vi "pseudoGellermann.vi"(11 "N":i32=10 min=10) -> (3 "Array":bool[](array[boolean]))   [LabVIEW 2013]
panel:
  out "Iterations":i32
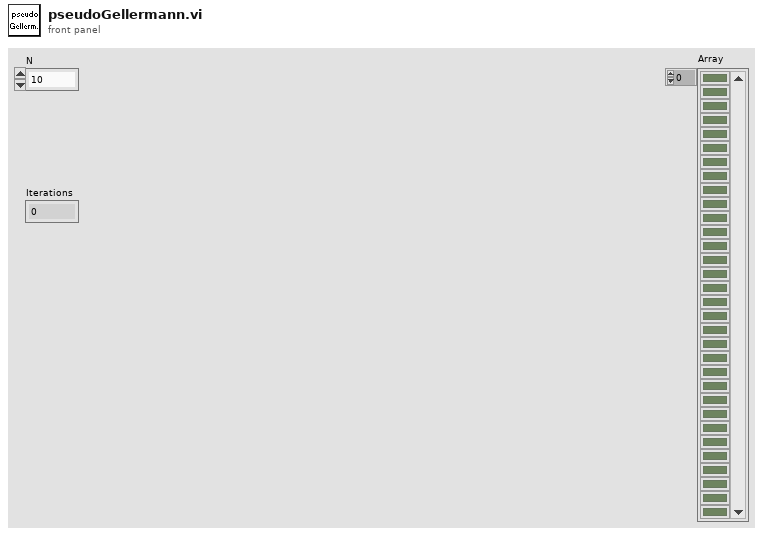
[diagram p1: front panel]
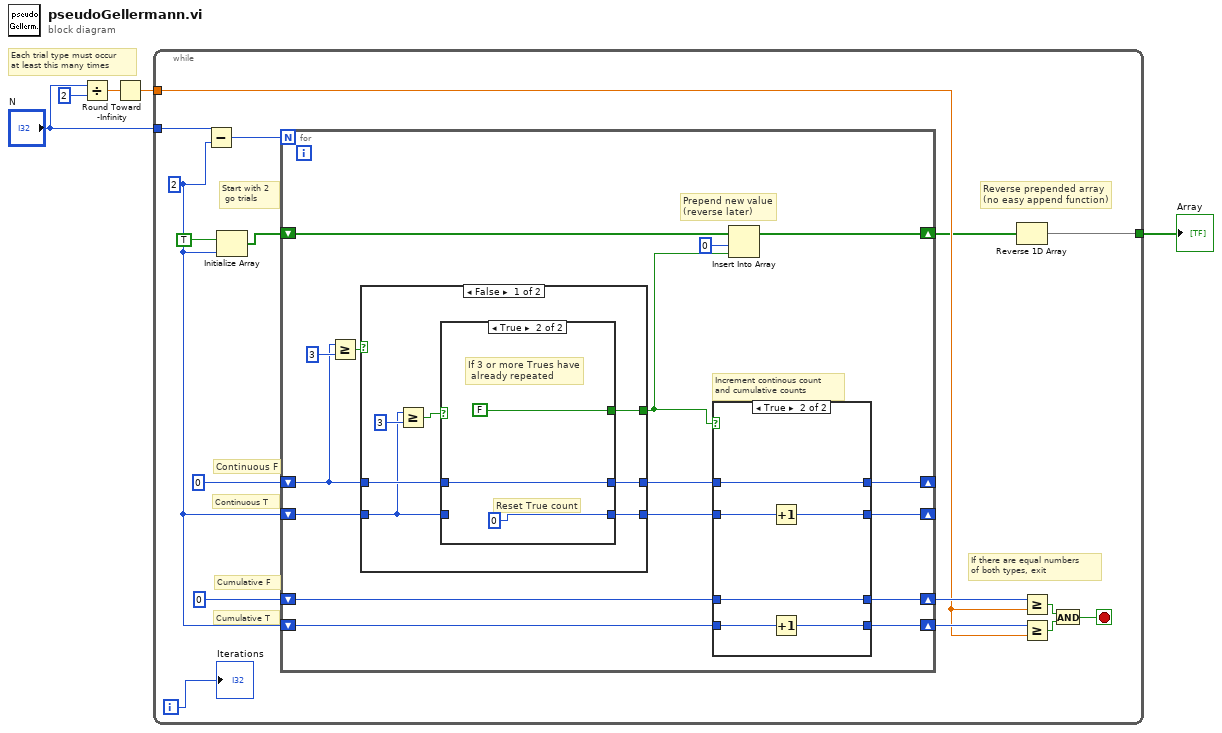
[diagram p0: block diagram]
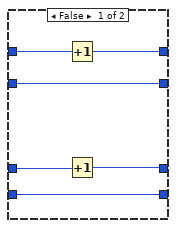
[diagram p2: hidden frame]
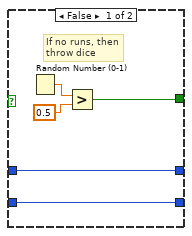
[diagram p3: hidden frame]
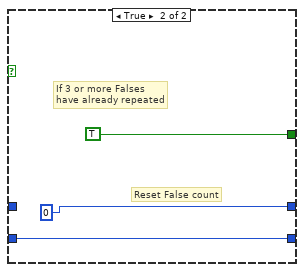
[diagram p4: hidden frame]
diagram:
  # "Each trial type must occur\nat least this many times"
  n1 = Divide(x="N", y=2) -> (x/y=w4:dbl)
  n2 = Round Toward -Infinity(1:w4) -> (0:w2:dbl)
  n3 = while {
    tunnel: "N" -> [w17]
    tunnel: w2 -> [w13]
    tunnel: [w8] -> w1
    i -> [w9]
    stop <- w10 stop-if-true
    w6 = 2 ("dimension size")
    # "Reverse prepended array\n(no easy append function)"
    # "If there are equal numbers\nof both types, exit"
    # "Cumulative T"
    # "Cumulative F"
    # "Start with 2\n go trials"
    # "Continuous T"
    # "Continuous F"
    n4 = Subtract(x=w17, y=w6) -> (x-y=w16:i32)
    n5 = Initialize Array(TRUE, w6) -> (w19:bool[])
    n6 = for {
      N: w16 -> [_]
      shift-right: [w23] -> _
      shift-left: 0 ("dimension size") -> [w35]
      shift-right: [w25] -> _
      shift-left: w6 -> [w34]
      shift-right: [w31] -> w7
      shift-left: w19 -> [w33]
      shift-right: [w28] -> w15
      shift-left: 0 ("dimension size") -> [w30]
      shift-right: [w27] -> w14
      shift-left: w6 -> [w29]
      # "Increment continous count\nand cumulative counts"
      # "Prepend new value\n(reverse later)"
      n7 = Greater Or Equal?(x=w35, y=3) -> (x >= y?=w37:bool)
      n8 = case shown="False" w37 {
        tunnel: w35 -> [w54 _]
        tunnel: w34 -> [w50 w66]
        tunnel: [w53 w66] -> w26
        tunnel: [w52 0 ("dimension size")] -> w24
        tunnel: [w51 TRUE] -> w22
        frame False {
          n9 = Greater Or Equal?(x=w50, y=3) -> (x >= y?=w55:bool)
          n10 = case shown="True" w55 {
            tunnel: w54 -> [w58 w63]
            tunnel: [w57 0 ("dimension size")] -> w53
            tunnel: [w58 w63] -> w52
            tunnel: [w59 FALSE] -> w51
            tunnel: w50 -> [w57 _]
            frame False {
              # "If no runs, then\nthrow dice"
              n11 = Random Number (0-1)() -> (number: 0 to 1=w61:dbl)
              n12 = Greater?(x=w61, y=0.5) -> (0:w59:bool)
            }
            frame True {
              # "Reset True count"
              # "If 3 or more Trues have\n already repeated"
            }
          }
        }
        frame True {
          # "Reset False count"
          # "If 3 or more Falses \nhave already repeated"
        }
      }
      n13 = case shown="True" w22 {
        tunnel: w30 -> [w40 w47]
        tunnel: w29 -> [w38 w49]
        tunnel: [w39 w47] -> w28
        tunnel: [w38 w48] -> w27
        tunnel: w26 -> [w41 w46]
        tunnel: [w41 w45] -> w25
        tunnel: w24 -> [w43 w44]
        tunnel: [w42 w44] -> w23
        frame False {
          n14 = Increment(x=w43) -> (x+1=w42:i32)
          n15 = Increment(x=w40) -> (x+1=w39:i32)
        }
        frame True {
          n16 = Increment(x=w46) -> (x+1=w45:i32)
          n17 = Increment(x=w49) -> (x+1=w48:i32)
        }
      }
      n18 = Insert Into Array(array=w33, index=0, new element=w22) -> (w31:bool[])
    }
    n19 = Reverse 1D Array(array=w7) -> (reversed array=w8:bool[])
    n20 = Greater Or Equal?(x=w15, y=w13) -> (x >= y?=w11:bool)
    n21 = Greater Or Equal?(x=w14, y=w13) -> (x >= y?=w12:bool)
    n22 = And(x=w11, y=w12) -> (x .and. y?=w10:bool)
    "Iterations" <- w9
  }
  "Array" <- w1
